vi "Control.vi"(3 "error in (no error)":errorcluster) -> (0 "error out":errorcluster)   [LabVIEW 2017]
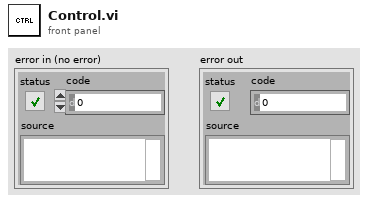
[diagram p1: front panel]
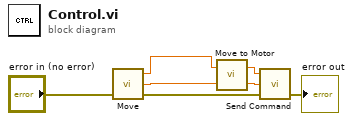
[diagram p0: block diagram]
diagram:
  n1 = call "Move.vi"("error in (no error)"="error in (no error)") -> ("error out"=w3:errorcluster, "Turn"=w2:dbl, "Forward"=w1:dbl)  [unwired: 2 in]
  n2 = call "Move to Motor.vi"("Turn"=w2, "Forward"=w1) -> ("Right"=w7:dbl, "Left"=w6:dbl)
  n3 = call "Send Command.vi"("error in (no error)"=w3, "Right"=w7, "Left"=w6) -> ("error out"=→"error out":errorcluster)  [unwired: 2 in]
